vi "Move Absolute.vi"(8 "error in (no error)":errorcluster, 9 "Desired Position":dbl, 10 "Axis Name":string, 11 "SIM Motion Controller in":refnum<class "SIM Motion Controller.lvclass">) -> (0 "error out":errorcluster, 3 "SIM Motion Controller out":refnum<class "SIM Motion Controller.lvclass">)   [LabVIEW 2022 SP3, in "SIM Motion Controller.lvclass"]
uses:
  SIM Motion Controller.lvclass
  SIM Motion Controller.lvclass/SIM Motion Controller.ctl
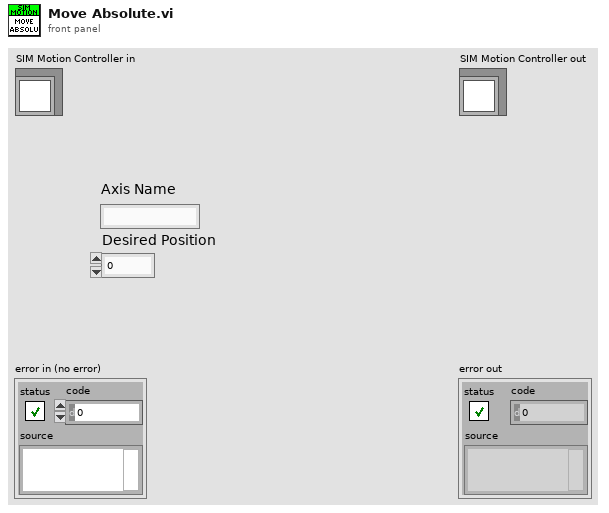
[diagram p1: front panel]
types:
  T1 = typedef "Motion Controller.lvclass/Axis Data.ctl" = cluster{"Axis Parameters":T2, "Axis Settings":T3}
  T2 = typedef "Motion Controller.lvclass/Axis Parameters.ctl" = cluster{"Moving":bool, "Homed":bool, "Desired Position":dbl, "Current Positon":dbl, "Current Speed":dbl}
  T3 = typedef "Motion Controller.lvclass/Axis Settings.ctl" = cluster{"Speed":dbl, "Acceleration":dbl}
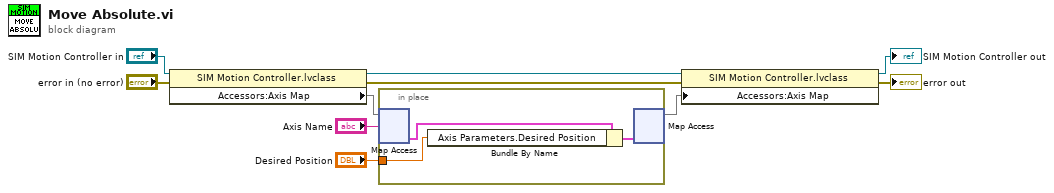
[diagram p0: block diagram]
diagram:
  n1 = property class="SIM Motion Controller.lvclass"(reference="SIM Motion Controller in", error in="error in (no error)") -> (reference out=w6:refnum<class "SIM Motion Controller.lvclass">, error out=w2:errorcluster, "Accessors:Axis Map"=w9:map{string, T1})
  n2 = in-place {
    in-place-border: "Desired Position" -> [w11]
    n3 = in-place-map #1(w9, "Axis Name") -> (w13:T1)  [unwired: 1 in, 1 out]
    n4 = Bundle By Name(cluster=w13, "Axis Parameters.Desired Position"=w11) -> (w12:T1)
    n5 = in-place-map #1(w12) -> (w7:map{string, T1})  [unwired: 1 in, 2 out]
  }
  n6 = property class="SIM Motion Controller.lvclass"(reference=w6, error in=w2, "Accessors:Axis Map"=w7) -> (reference out=→"SIM Motion Controller out":refnum<class "SIM Motion Controller.lvclass">, error out=→"error out":errorcluster)
